vi "Diddle RTS.vi"(8 "error in (no error)":errorcluster) -> (0 "error out":errorcluster, 3 "CTS off?":bool)   [LabVIEW 2013]
uses:
  NanoArduino/NanoCmds.ctl
  <vilib>/Instr/_visa.llb/VISA Configure Serial Port (Instr).vi
panel:
  out "CTS on?":bool
  out "Read Value 2":dbl
  out "Read Value":dbl
  out "read buffer":string
  in  "VISA resource name":refnum<visa-resource-name>="COM30"
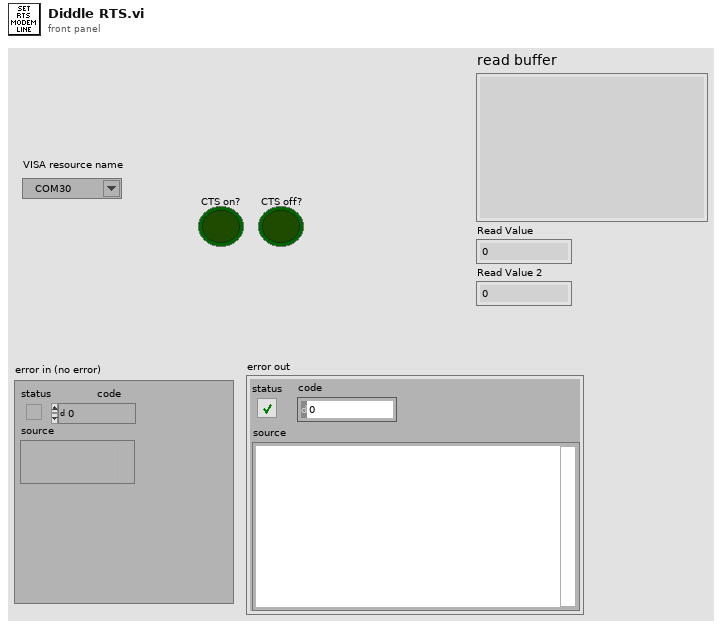
[diagram p1: front panel]
types:
  T1 = typedef "NanoCmds.ctl" = enum16{"Make digital port an output", "Make digital port an input", "Set digital pin high", "Set digital pin low", "Get digital pin state", "Get analog pin voltage", "Get analog pins difference", "Get ohms at analog pin", "Turn on current limit", "Reset Nano device", "Get digital pin state pullup", "Read current", "Initialize", "Power up uut", "Power down uut", "Get uut current draw", "Set ADC volts high", "Set ADC volts low", "Start up uut modem", "Get CTS state", "Get on_nsleep state", "Reset modem", "Get lid state", "Wait for lid closed", "Wait for lid open", "Power up, start, get curr", "Check if X2 shorted", "Power up and start up", "Check X3 shorted"}
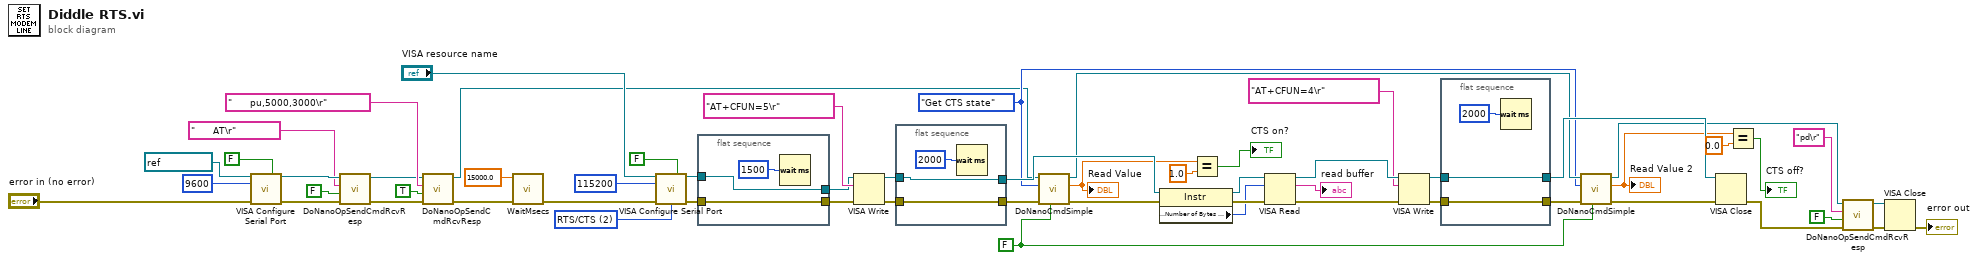
[diagram p0: block diagram]
diagram:
  w30 = FALSE ("SerialNotOpen?")
  w32 = NanoCmds."Get CTS state" ("Nano Op")
  w58 = u16 2 items=["None", "XON/XOFF", "RTS/CTS", "XON/XOFF & RTS/CTS", "DTR/DSR", "XON/XOFF & DTR/DSR"] ("flow control (0:none)")
  n1 = call-poly "VISA Configure Serial Port"("VISA resource name"=refnum<visa-resource-name> "COM21", "Enable Termination\nChar (T)"=FALSE ("Enable Termination\nChar (T)"), "baud rate (9600)"=u32 9600, "error in (no error)"="error in (no error)") -> ("VISA resource name out"=w9:refnum<visa-resource-name>, "error out"=w11:errorcluster)  [unwired: 10 in]
  n2 = call "DoNanoOpSendCmdRcvResp.vi"("error in (no error)"=w11, "Wait after response"=FALSE, "Cmd String"="      AT\r", "VISA resource name"=w9) -> ("error out"=w10:errorcluster, "VISA resource name out"=w8:refnum<visa-resource-name>)  [unwired: 1 in, 5 out]
  n3 = call "DoNanoOpSendCmdRcvResp.vi"("error in (no error)"=w10, "Wait after response"=TRUE, "Cmd String"="      pu,5000,3000\r", "VISA resource name"=w8) -> ("error out"=w15:errorcluster, "VISA resource name out"=w17:refnum<visa-resource-name>)  [unwired: 1 in, 5 out]
  n4 = call "WaitMsecs.vi"("error in (no error)"=w15, "Wait Msecs"=15000.0) -> ("error out"=w13:errorcluster)  [unwired: 9 in]
  n5 = call-poly "VISA Configure Serial Port"("VISA resource name"="VISA resource name", "Enable Termination\nChar (T)"=FALSE ("Enable Termination\nChar (T)"), "baud rate (9600)"=u32 115200, "error in (no error)"=w13, "flow control (0:none)"=w58) -> ("VISA resource name out"=w48:refnum<visa-resource-name>, "error out"=w49:errorcluster)  [unwired: 9 in]
  n6 = flat-sequence {
    tunnel: w48 -> [w60]
    tunnel: w49 -> [w59]
    tunnel: [w60] -> w47
    tunnel: [w59] -> w46
    frame #0 {
      n7 = Wait (ms)(milliseconds to wait=u32 1500) -> ()  [unwired: 1 out]
    }
  }
  n8 = VISA Write(VISA resource name=w47, write buffer="AT+CFUN=5\r", error in (no error)=w46) -> (VISA resource name out=w55:refnum<visa-resource-name>, error out=w54:errorcluster)  [unwired: 1 out]
  n9 = flat-sequence {
    tunnel: w55 -> [w63]
    tunnel: w54 -> [w62]
    tunnel: [w63] -> w36
    tunnel: [w62] -> w38
    frame #0 {
      n10 = Wait (ms)(milliseconds to wait=u32 2000) -> ()  [unwired: 1 out]
    }
  }
  n11 = call "DoNanoCmdSimple.vi"("SerialNotOpen?"=w30, "error in (no error)"=w38, "Nano Op"=w32, "VISA resource name"=w17) -> ("error out"=w37:errorcluster, "Read Value"=w25:dbl, "VISA resource name 2"=w33:refnum<visa-resource-name>)  [unwired: 3 in, 1 out]
  "Read Value" <- w25
  n12 = property class="Instr"(reference=w36, error in=w37) -> (reference out=w53:refnum<visa-resource-name>, error out=w52:errorcluster, "Serial Settings:Number of Bytes at Serial Port"=w51:u32)
  n13 = Equal?(x=w25, y=1.0) -> (x = y?=→"CTS on?":bool)
  n14 = VISA Read(VISA resource name=w53, byte count=w51, error in (no error)=w52) -> (VISA resource name out=w42:refnum<visa-resource-name>, read buffer=→"read buffer":string, error out=w43:errorcluster)  [unwired: 1 out]
  n15 = VISA Write(VISA resource name=w42, write buffer="AT+CFUN=4\r", error in (no error)=w43) -> (VISA resource name out=w39:refnum<visa-resource-name>, error out=w40:errorcluster)  [unwired: 1 out]
  n16 = flat-sequence {
    tunnel: w39 -> [w66]
    tunnel: w40 -> [w65]
    tunnel: [w66] -> w34
    tunnel: [w65] -> w35
    frame #0 {
      n17 = Wait (ms)(milliseconds to wait=u32 2000) -> ()  [unwired: 1 out]
    }
  }
  n18 = call "DoNanoCmdSimple.vi"("SerialNotOpen?"=w30, "error in (no error)"=w35, "Nano Op"=w32, "VISA resource name"=w33) -> ("error out"=w31:errorcluster, "Read Value"=w29:dbl, "VISA resource name 2"=w5:refnum<visa-resource-name>)  [unwired: 3 in, 1 out]
  "Read Value 2" <- w29
  n19 = VISA Close(VISA resource name=w34, error in (no error)=w31) -> (error out=w3:errorcluster)
  n20 = Equal?(x=w29, y=0.0) -> (x = y?=→"CTS off?":bool)
  n21 = call "DoNanoOpSendCmdRcvResp.vi"("error in (no error)"=w3, "Wait after response"=FALSE, "Cmd String"="pd\r", "VISA resource name"=w5) -> ("error out"=w2:errorcluster, "VISA resource name out"=w1:refnum<visa-resource-name>)  [unwired: 1 in, 5 out]
  n22 = VISA Close(VISA resource name=w1, error in (no error)=w2) -> (error out=→"error out":errorcluster)
